vi "Read Timeout.vi"(8 "error in (no error)":errorcluster, 11 "Dialog.lvclass in":refnum<class "Dialog.lvclass">) -> (0 "error out":errorcluster, 2 "Timeout":i32=-1, 3 "Dialog.lvclass out":refnum<class "Dialog.lvclass">)   [LabVIEW 2012, in "Dialog.lvlib" / "Dialog.lvclass"]
doc: "Accessor VI for Dialog class."
uses:
  Dialog.lvclass
  Dialog.lvclass/Dialog.ctl
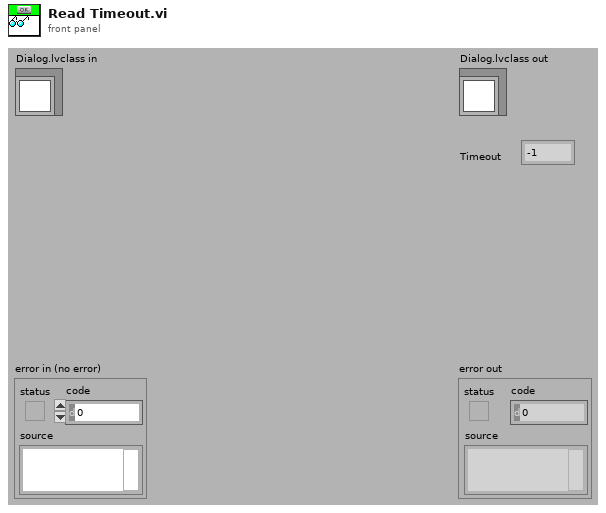
[diagram p1: front panel]
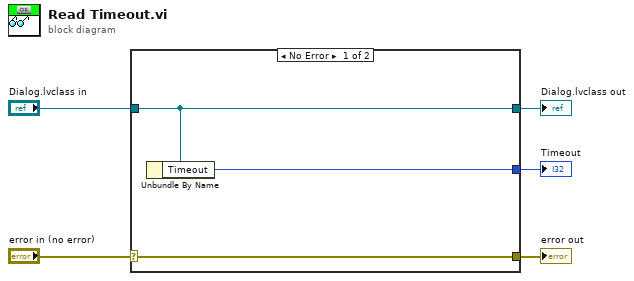
[diagram p0: block diagram]
diagram:
  n1 = case shown="No Error" "error in (no error)" {
    selector: "error in (no error)" -> [w8 w9]
    tunnel: [w8 w9] -> w4
    tunnel: [w7 w10] -> w2
    tunnel: "Dialog.lvclass in" -> [w7 w10]
    tunnel: [w6 _] -> w1
    frame No Error {
      n2 = Unbundle By Name(w7) -> ("Timeout"=w6:i32)
    }
    frame Error {
    }
  }
  "error out" <- w4
  "Dialog.lvclass out" <- w2
  "Timeout" <- w1
